vi "apply modification.vi"(10 "vis":refnum<vi>[](array[refnum]), 11 "control label adjustment in":refnum<class "control label adjustment.lvclass">) -> (0 "error report":errorcluster[](array[cluster]), 3 "control label adjustment out":refnum<class "control label adjustment.lvclass">)   [LabVIEW 2013, in "control label adjustment.lvclass"]
uses:
  control label adjustment.lvclass
  control label adjustment.lvclass/control label adjustment.ctl
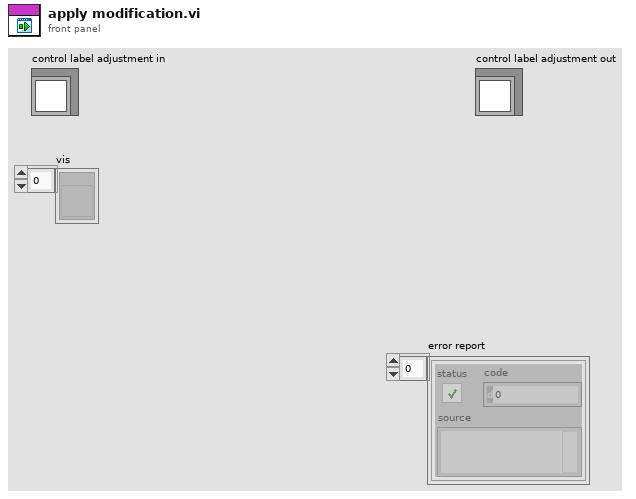
[diagram p1: front panel]
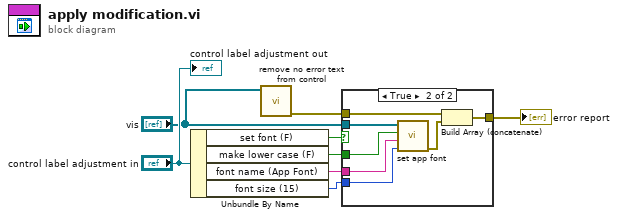
[diagram p0: block diagram]
diagram:
  n1 = Unbundle By Name("control label adjustment in") -> ("set font (F)"=w7:bool, "make lower case (F)"=w3:bool, "font name (App Font)"=w1:string, "font size (15)"=w2:u32)
  n2 = call "remove no error text from control.vi"("vis"="vis") -> ("error report"=w5:errorcluster[])  [unwired: 10 in]
  n3 = case shown="True" w7 {
    tunnel: [w9 w14] -> w6
    tunnel: w5 -> [w9 w16]
    tunnel: "vis" -> [_ w13]
    tunnel: w3 -> [_ w12]
    tunnel: w2 -> [_ w11]
    tunnel: w1 -> [_ w10]
    frame False {
    }
    frame True {
      n4 = call "set app font.vi"("font size"=w11, "font name (App Font)"=w10, "make lower case"=w12, "vis"=w13) -> ("error report"=w15:errorcluster[])  [unwired: 7 in]
      n5 = Build Array (concatenate)(w16, w15) -> (w14:errorcluster[])
    }
  }
  "error report" <- w6
  "control label adjustment out" <- "control label adjustment in"
